vi "calculate channel change.vi"(1 "set index":i32, 4 "Location Cluster in":T1) -> (14 "action":string, 16 "keystrokes":string, 18 "rows difference":i32)   [LabVIEW 2018]
uses:
  location cluster.ctl
  CAEN globals.vi
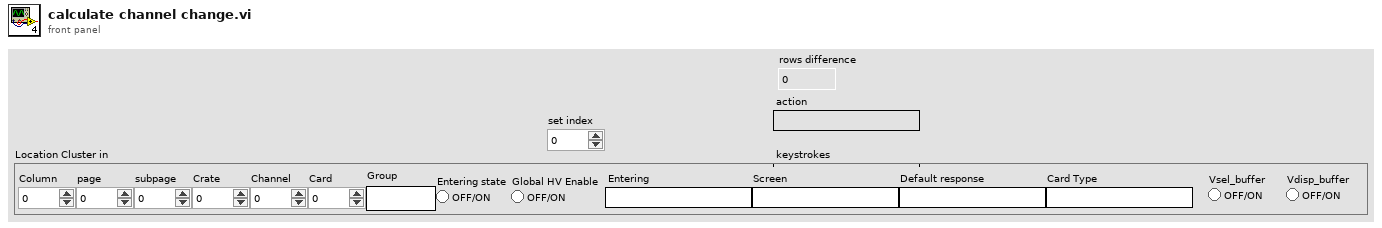
[diagram p1: front panel]
types:
  T1 = typedef "location cluster.ctl" = cluster{"Column":i32, "Card Type":string, "Channel":i32, "Card":i32, "Default response":string, "Entering":string, "Entering state":bool, "subpage":i32, "page":i32, "Crate":i32, "Screen":string, "Group":string, "Global HV Enable":bool, "Vsel_buffer":bool, "Vdisp_buffer":bool}
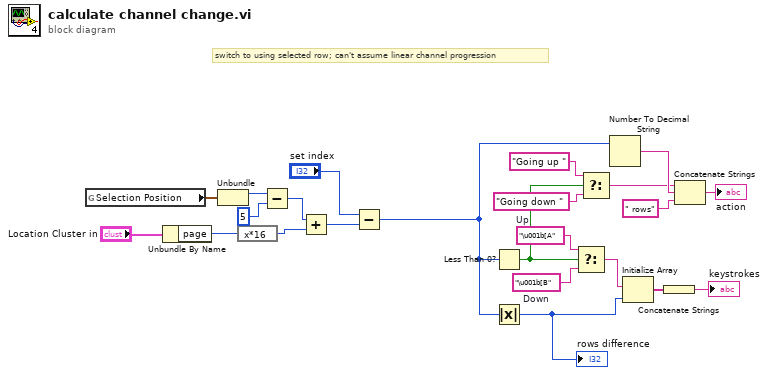
[diagram p0: block diagram]
diagram:
  w11 = "\u001b[A"  # Up
  w10 = "\u001b[B"  # Down
  # "switch to using selected row; can't assume linear channel progression"
  n1 = global read "CAEN globals.vi" "Selection Position"() -> (w8:cluster{i32, i32})
  n2 = Unbundle By Name("Location Cluster in") -> ("page"=w1:i32)
  n3 = Unbundle(w8) -> (w7:i32)  [unwired: 1 out]
  n4 = expression code="x*16"(w1) -> (w5:i32)
  n5 = Subtract(x=w7, y=5) -> (x-y=w4:i32)
  n6 = Add(x=w4, y=w5) -> (x+y=w3:i32)
  n7 = Subtract(x="set index", y=w3) -> (x-y=w19:i32)
  n8 = Less Than 0?(x=w19) -> (x < 0?=w17:bool)
  n9 = Absolute Value(x=w19) -> (abs(x)=w15:i32)
  "rows difference" <- w15
  n10 = Select(t=w11, s=w17, f=w10) -> (s? t:f=w12:string)
  n11 = Select(t="Going up " ("Up"), s=w17, f="Going down " ("Down")) -> (s? t:f=w20:string)
  n12 = Number To Decimal String(number=w19) -> (decimal integer string=w21:string)  [unwired: 1 in]
  n13 = Initialize Array(w12, w15) -> (w13:string[])
  n14 = Concatenate Strings(w13) -> (→"keystrokes":string)
  n15 = Concatenate Strings(w20, w21, " rows" ("Down")) -> (→"action":string)
